vi "Get Path Regex.vi"(8 "error in (no error)":errorcluster, 11 "Controller in":refnum<class "Controller.lvclass">) -> (0 "error out":errorcluster, 2 "Path Regex":string, 3 "Controller out":refnum<class "Controller.lvclass">)   [LabVIEW 2020, in "HTTP Server.lvlib" / "Controller.lvclass"]
doc: "Specifies the request path that the controller handles requests for in the form of a PCRE regular expression and uses LabVIEW's Match Regular Expression functionality (but not the XNode). Since this uses regular expressions there are some common tricks to avoid odd behavior that might be seen with longer paths that have repeated segments. Eventually the plan is to provide an API that can help build the desired regular expressions but for now you'll need to understand the quirks they can bring.\n\nAll request paths start with \"/\" and to ensure your desired path matches from the start of the request path, put a \"^\" at the beginning. For example, a pattern of \"/test\" could match \"/test/foo\", \"/test\", \"/foo/test\", and many more. To ensure the URL begins with \"/test\" use a pattern of \"^/test\".\n\nSimilar to anchoring a match to the start of the path, the match can be anchored to the end of the path as well with \"$\" added to the end. For example, \"^/test$\" would match exactly \"/test\" and nothing else while a pattern of \"/test$\" would match \"/test\", \"/foo/test\", \"/bar/test\" and anything ending with \"/test\".\n\nSubmatches are also handled and can allow for segments of the path to become variables that are retrievable from the processing values container. As an example \"^/test/(\\d+)$\" would match any url starting with \"/test/\" followed by a number, such as when requesting a test ID to be viewed from a database. Submatches are put into the values container in the same order they'd be returned from the Match Regular Expression node with a lookup value of the string representation of the value's 0-based index. To continue the /test/# example from above, the numeric value part of the path could be retrieved by calling Get Value by Name.vi with a name of \"0\". Values are returned as a variant and will need to be converted to the appropriate type. Since paths are string values, the variant will first need to be converted back into a string and can then be converted from the string to intended final data type.\n\nAnother submatch example: \"^/post/(\\d+)/comment/(\\d+)$\" which provides two submatches. The post ID would be retrieved with a name of \"0\" and the comment ID with a name of \"1\"."
uses:
  Controller.lvclass
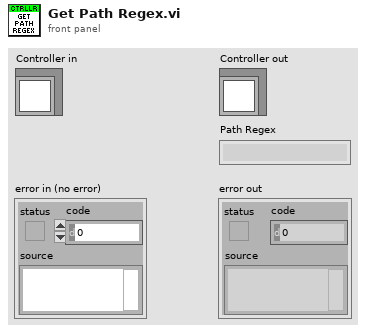
[diagram p1: front panel]
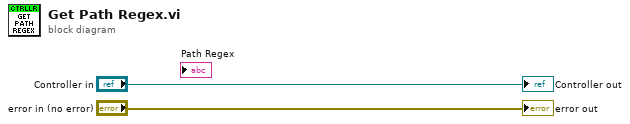
[diagram p0: block diagram]
diagram:
  "error out" <- "error in (no error)"
  "Controller out" <- "Controller in"
